vi "方程事件2.vi"() -> ()   [LabVIEW 2018]
panel:
  in  "计算":bool
  out "结果":dbl
  in  "C":dbl
  in  "B":dbl
  in  "X":dbl
  in  "A":dbl
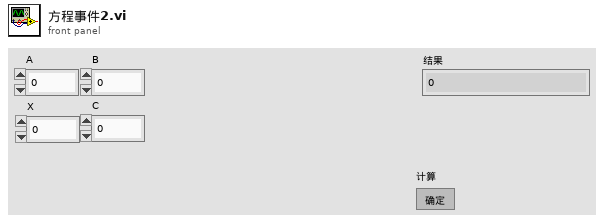
[diagram p1: front panel]
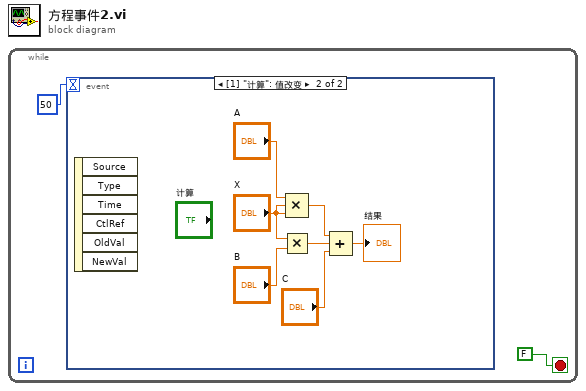
[diagram p0: block diagram]
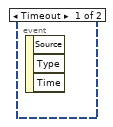
[diagram p2: hidden frame]
diagram:
  n1 = while {
    stop <- FALSE stop-if-true
    n2 = event shown="[1] \"计算\": 值改变" {
      selector: _ -> [_ _]
      dyn-events: _ -> [_ _]
      timeout: 50 -> [_ _]
      event Timeout {
        n3 = event-data() -> ()  [unwired: 1 in, 3 out]
      }
      event "计算": Value Change {
        n4 = event-data() -> ()  [unwired: 1 in, 6 out]
        n5 = Multiply(x="X", y="B") -> (x*y=w8:dbl)
        n6 = Compound Arithmetic op=MULTIPLY("A", "X", "X") -> (w7:dbl)
        n7 = Compound Arithmetic op=ADD(w7, w8, "C") -> (→"结果":dbl)
      }
    }
  }
